vi "Overlay.vi"(8 "error in (no error)":errorcluster, 10 "Image In":T1, 11 "Overlay Base in":refnum<class "Analyze Results Beam Deviation.lvclass">) -> (0 "error out":errorcluster, 2 "Image out":T1, 3 "Overlay Base out":refnum<class "Analyze Results Beam Deviation.lvclass">)   [LabVIEW 2014, in "Analyze Results Beam Deviation.lvclass"]
uses:
  Analyze Results Beam Deviation.lvclass
  <vilib>/vision/Image Controls.llb/IMAQ Image.ctl
  Analyze Results Beam Deviation.lvclass/Analyze Results Beam Deviation.ctl
  Results Base/Analyze Results Base.lvclass/Analyze Results Base.ctl
  Results Base/Read Overlay_.vi
  Results Base/Read Overlay colors.vi
  Results Base/Read Font, Size & Style.vi
  Results Base/Read Position.vi
  Results Base/Analyze Results Base.lvclass
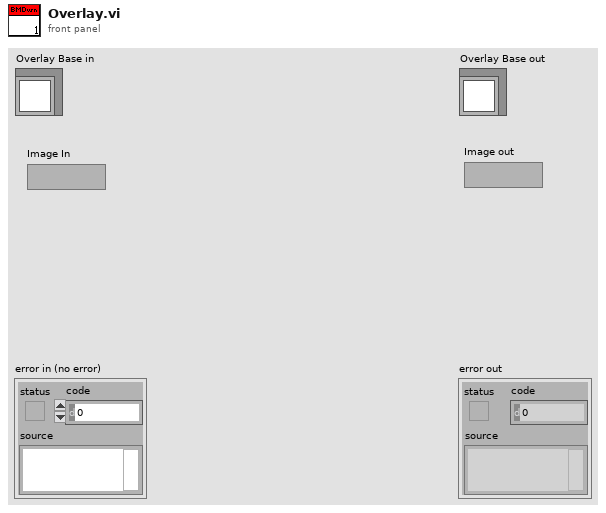
[diagram p1: front panel]
types:
  T1 = typedef "IMAQ Image.ctl" = refnum<image>
  T2 = cluster{"Desired Font (Application)":enum16{"User-specified Font", "Application Font", "System Font", "Dialog Font"}, "[User-specified Font]":cluster{"Font Name":string, "Size":i16, "Strikeout?":bool, "Italic?":bool, "Underline?":bool, "Outline?":bool, "Shadow?":bool, "Bold?":bool, "Rotation Angle":dbl}, "Horizontal Alignment":i16, "Vertical Alignment":i16}
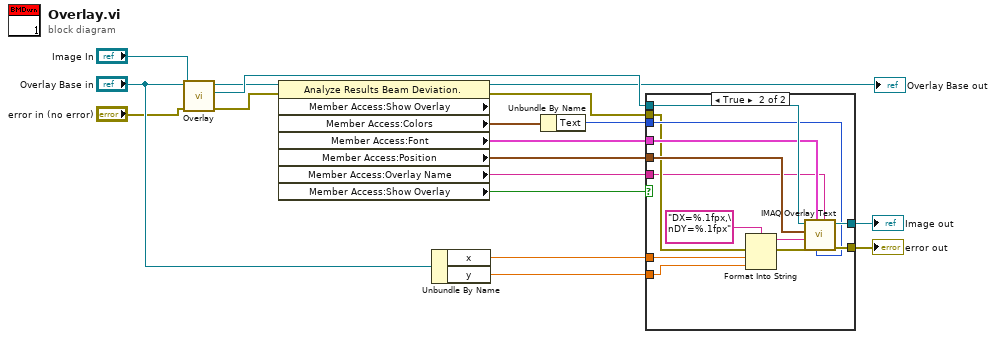
[diagram p0: block diagram]
diagram:
  n1 = call-parent "Overlay.vi"("error in (no error)"="error in (no error)", "Image In"="Image In", "Overlay Base in"="Overlay Base in") -> ("error out"=w3:errorcluster, "Image out"=w14:T1, "Overlay Base out"=w5:refnum<class "Analyze Results Beam Deviation.lvclass">)  [unwired: 6 in]
  n2 = property class="Analyze Results Beam Deviation." props=["Member Access:Show Overlay", "Member Access:Colors", "Member Access:Font", "Member Access:Position", "Member Access:Overlay Name", "Member Access:Show Overlay"](reference=w5, error in=w3) -> (reference out=→"Overlay Base out":refnum<class "Analyze Results Beam Deviation.lvclass">, error out=w2:errorcluster, "Member Access:Colors"=w11:cluster{"Border":u32, "Text":u32}, "Member Access:Font"=w9:T2, "Member Access:Position"=w8:cluster{"x":i16, "y":i16}, "Member Access:Overlay Name"=w18:string, "Member Access:Show Overlay"=w7:bool)  [unwired: 1 out]
  n3 = Unbundle By Name("Overlay Base in") -> ("x"=w13:dbl, "y"=w12:dbl)
  n4 = Unbundle By Name(w11) -> ("Text"=w10:u32)
  n5 = case shown="True" w7 {
    tunnel: w14 -> [w20 w33]
    tunnel: [w20 w32] -> w15
    tunnel: [w19 w31] -> w16
    tunnel: w2 -> [w19 w25]
    tunnel: w13 -> [_ w27]
    tunnel: w12 -> [_ w26]
    tunnel: w10 -> [_ w30]
    tunnel: w9 -> [_ w29]
    tunnel: w8 -> [_ w28]
    tunnel: w18 -> [_ w21]
    frame False {
    }
    frame True {
      n6 = Format Into String(format string="DX=%.1fpx,\nDY=%.1fpx", error in=w25, w27, w26) -> (resulting string=w24:string, error out=w23:errorcluster)  [unwired: 1 in]
      n7 = call "IMAQ Overlay Text"("Group"=w21, "Text Color (black)"=w30, "Font, Size & Style"=w29, "error in (no error)"=w23, "String"=w24, "Origin"=w28, "Image"=w33) -> ("error out"=w31:errorcluster, "Image Out"=w32:T1)  [unwired: 3 in]
    }
  }
  "error out" <- w16
  "Image out" <- w15
